vi "Test Get Output.vi"() -> ()   [LabVIEW 2016, in "Spectrum Recorder.lvclass"]
uses:
  Spectrum Recorder.lvclass
  Spectrum Recorder.lvclass/Spectrum Recorder.ctl
panel:
  out "size(s)":i32
  out "Output values out":dbl[](array[numeric])
  out "Waveform Graph":dbl[](graph)
  in  "Number of points":i32=100
  in  "User Configuration.Repeat (-1: forever)":i32=1
  in  "Output counter":i32
  in  "Records counter":i32
  in  "Output values in":dbl[](array[numeric])=[1.0, 2.0, 3.0, 4.0, 5.0, 6.0, 7.0, 8.0, 9.0, 10.0]
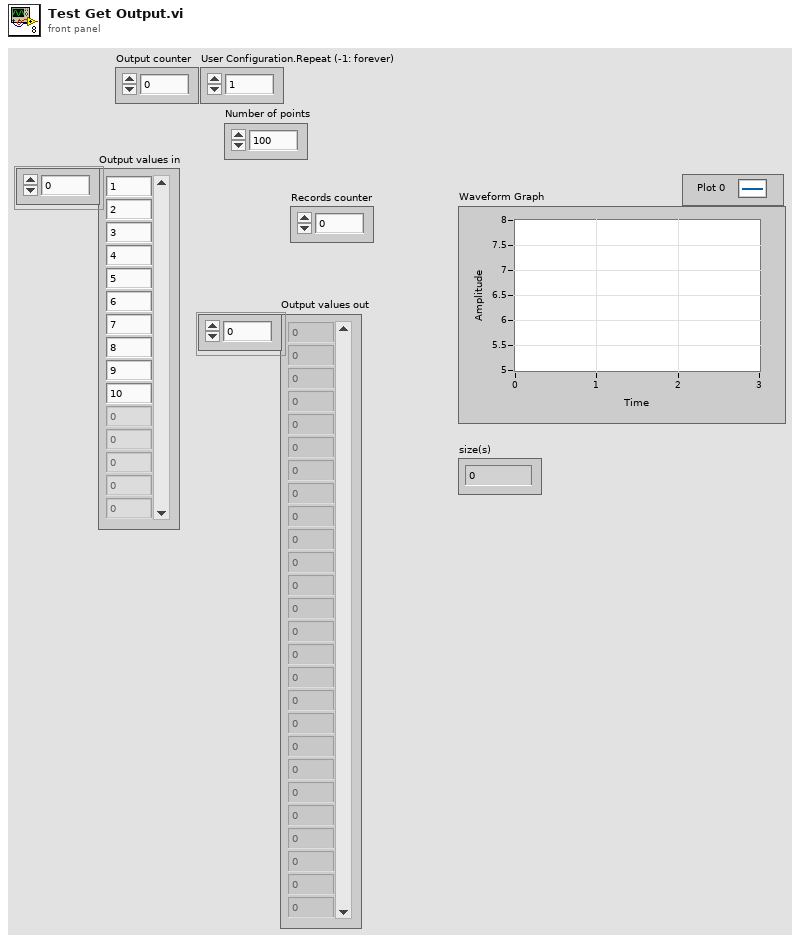
[diagram p1: front panel]
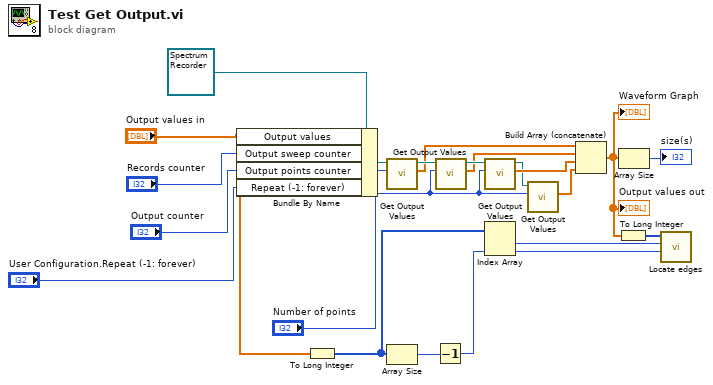
[diagram p0: block diagram]
diagram:
  n1 = Bundle By Name(cluster=refnum<class "Spectrum Recorder.lvclass"> refnum ("Spectrum Recorder.lvclass"), "Output values"="Output values in", "Output sweep counter"="Records counter", "Output points counter"="Output counter", "Repeat (-1: forever)"="User Configuration.Repeat (-1: forever)") -> (w18:refnum<class "Spectrum Recorder.lvclass">)
  n2 = To Long Integer(number="Output values in") -> (32bit integer=w2:i32[])
  n3 = call-dynamic "Get Output Values.vi"("Number of points"="Number of points", "Spectrum Recorder in"=w18) -> ("Output values"=w14:dbl[], "Spectrum Recorder out"=w16:refnum<class "Spectrum Recorder.lvclass">)  [unwired: 7 in, 1 out]
  n4 = Array Size(array=w2) -> (size(s)=w7:i32)
  n5 = Decrement(x=w7) -> (x-1=w6:i32)
  n6 = call-dynamic "Get Output Values.vi"("Number of points"="Number of points", "Spectrum Recorder in"=w16) -> ("Output values"=w13:dbl[], "Spectrum Recorder out"=w15:refnum<class "Spectrum Recorder.lvclass">)  [unwired: 7 in, 1 out]
  n7 = call-dynamic "Get Output Values.vi"("Number of points"="Number of points", "Spectrum Recorder in"=w15) -> ("Output values"=w12:dbl[], "Spectrum Recorder out"=w11:refnum<class "Spectrum Recorder.lvclass">)  [unwired: 7 in, 1 out]
  n8 = Index Array(array=w2, index #2=w6) -> (element #1=w5:i32, element #2=w4:i32)  [unwired: 1 in]
  n9 = call-dynamic "Get Output Values.vi"("Number of points"="Number of points", "Spectrum Recorder in"=w11) -> ("Output values"=w9:dbl[])  [unwired: 7 in, 2 out]
  n10 = Build Array (concatenate)(w14, w13, w12, w9) -> (w8:dbl[])
  "Waveform Graph" <- w8
  "Output values out" <- w8
  n11 = To Long Integer(number=w8) -> (32bit integer=w1:i32[])
  n12 = Array Size(array=w8) -> (size(s)=→"size(s)":i32)
  n13 = call "Locate edges.vi"("Last value"=w4, "First value"=w5, "Values"=w1) -> ()  [unwired: 7 in, 2 out]
